vi "Periodic Tasks.vi"(8 "error in":errorcluster) -> ()   [LabVIEW 2012]
doc: "This VI runs in parallel to other tasks. It can contain as many user-defined periodic loops as you need. These can carry out PID or other sorts of timed response."
uses:
  <vilib>/Rock Robotics/WPI/DriverStation/DriverStationLCD/WPI_DriverStationLCDLCDLine.ctl
  <vilib>/Rock Robotics/SystemInterfaces/Utilities/FPGA_UtilitiesLED Source.ctl
  <vilib>/Rock Robotics/SystemInterfaces/Utilities/FPGA_UtilitiesLED State.ctl
  Robot Global Data.vi
  <vilib>/Rock Robotics/Network Tables/SD Write Boolean.vi
  <vilib>/Rock Robotics/Network Tables/SD Write Number.vi
  <vilib>/Rock Robotics/WPI/Solenoid/Deprecated/WPI_SolenoidSetBool.vi
  <vilib>/Rock Robotics/WPI/Solenoid/Deprecated/WPI_SolenoidGetBool.vi
  <vilib>/Rock Robotics/WPI/Compressor/WPI_CompressorGetSetRefNum.vi
  <vilib>/Rock Robotics/SystemInterfaces/Typedef/FPGA_TypedefAnalogModule.ctl
panel:
  out "Value":bool
  out "Up?":bool
  in  "Holding Force":dbl=0.75
  in  "Desired Speed":dbl=9500.0
  in  "Cam Speed":dbl=1.0
  out "Up to Speed?":bool
  in  "Minimum Speed":dbl=9500.0
  in  "Low Stop-Band":dbl=6.0
  in  "Scalar Multiplier":dbl=0.08
  in  "High Stop-Band":dbl=1.5
  in  "In Deadband Strength":dbl=0.5
  in  "Angle Based Deadband":dbl=7.0
  in  "PID Vision gains":T1={"proportional gain (Kc)"=1.1, "integral time (Ti, min)"=0.0, "derivative time (Td, min)"=0.0}
  in  "PID gains":T1={"proportional gain (Kc)"=0.165, "integral time (Ti, min)"=0.0, "derivative time (Td, min)"=0.0}
  in  "Teleop Vision Offset":dbl=-0.62
  in  "Autonomous Vision Offset":dbl=-0.505
  out "RPM":dbl
  in  "Voltage Adjustment":dbl=12.0
  out "Adjusted For Voltage":dbl
  out "robot battery voltage":dbl
  out "Shooter Rotation Angle":dbl
  in  "OversampleBits":u8=1
  in  "Update Averaging And Stuff":bool
  in  "AverageBits":u8
  in  "Samples Per Second":dbl
  in  "Update Sampling Rate":bool
  # "In Automatic Mode, the hopper runs unless all beam sensors are tripped. This needs refining-\nit drains batterey. Once we figure out how to best control the shooter, we can tell it to run when \nwe want to intake from the feeder station and when we want to shoot and have a fourth disk still in the belts."
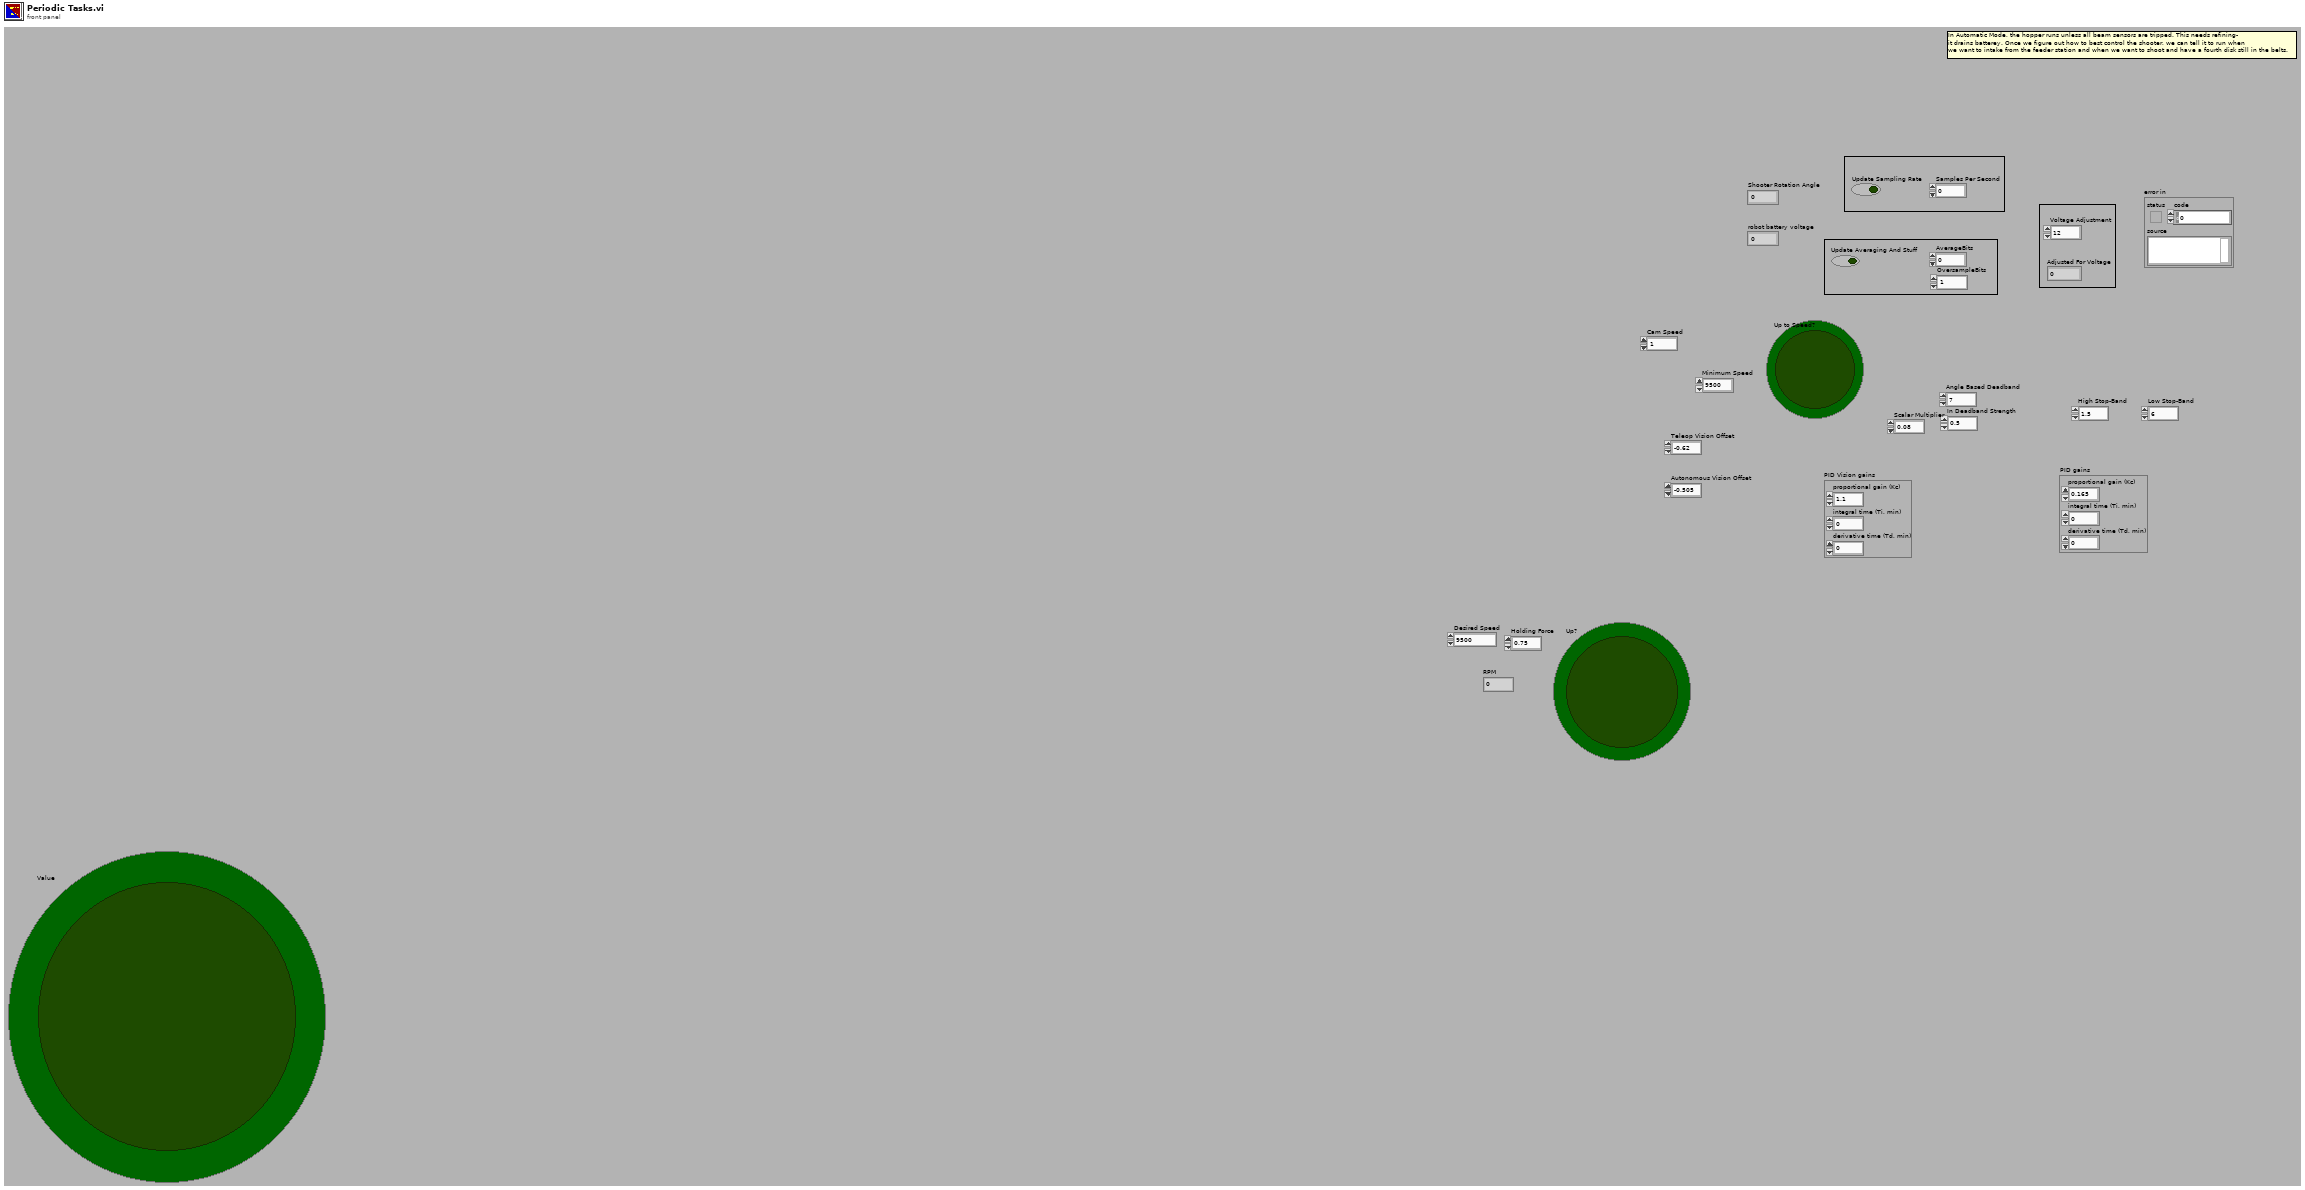
[diagram p1: front panel]
types:
  T1 = cluster{"proportional gain (Kc)":dbl, "integral time (Ti, min)":dbl, "derivative time (Td, min)":dbl}
  T2 = typedef "WPI_AnalogChannelDevRef.ctl" = cluster{"DevStatus":errorcluster, "Analog Module":T3, "Analog Channel":T4}
  T3 = typedef "FPGA_TypedefAnalogModule.ctl" = enum16{"Analog Module 1", "Analog Module 2"}
  T4 = typedef "FPGA_AIChannel.ctl" = enum8{"AI 1", "AI 2", "AI 3", "AI 4", "AI 5", "AI 6", "AI 7", "AI 8", "Invalid"}
  T5 = typedef "WPI_CounterDevRef.ctl" = cluster{"DevStatus":errorcluster, "CntIndex":T6}
  T6 = typedef "FPGA_CounterCtrSystemIndex.ctl" = enum8{"Ctr 0", "Ctr 1", "Ctr 2", "Ctr 3", "Ctr 4", "Ctr 5", "Ctr 6", "Ctr 7", "Invalid"}
  T7 = typedef "FPGA_UtilitiesLED State.ctl" = enum16{"Off", "On", "Toggle"}
  T8 = typedef "FPGA_UtilitiesLED Source.ctl" = enum16{"User LED", "FPGA LED"}
  T9 = typedef "WPI_DriverStationLCDLCDLine.ctl" = enum16{"Main - Line 1", "User - Line 2", "User - Line 3", "User - Line 4", "User - Line 5", "User - Line 6"}
  T10 = typedef "WPI_CompressorDevRef.ctl" = cluster{"DevStatus":errorcluster, "DigitalInputDevRef":T11, "RelayDevRef":T14}
  T11 = typedef "WPI_DigitalInputDevRef.ctl" = cluster{"DevStatus":errorcluster, "DIO Channel":T12, "Digital Module":T13}
  T12 = typedef "FPGA_DIOChannel.ctl" = enum8{"DIO 1", "DIO 2", "DIO 3", "DIO 4", "DIO 5", "DIO 6", "DIO 7", "DIO 8", "DIO 9", "DIO 10", "DIO 11", "DIO 12", "DIO 13", "DIO 14", "Invalid"}
  T13 = typedef "FPGA_TypedefDigitalModule.ctl" = enum16{"Digital Module 1", "Digital Module 2"}
  T14 = typedef "WPI_RelayDevRef.ctl" = cluster{"DevStatus":errorcluster, "Relay Channel":T15, "Digital Module":T13, "Relay Direction":T16}
  T15 = typedef "FPGA_DIORelayChannel.ctl" = enum8{"Relay 1", "Relay 2", "Relay 3", "Relay 4", "Relay 5", "Relay 6", "Relay 7", "Relay 8", "Invalid"}
  T16 = typedef "WPI_RelayDirection.ctl" = enum16{"Both directions", "Forward only", "Reverse only"}
  T17 = typedef "WPI_SolenoidDevRef.ctl" = cluster{"DevStatus":errorcluster, "Solenoid Module":T18, "Forward Solenoid Channel":T19, "Reverse Solenoid Channel":T19}
  T18 = typedef "FPGA_TypedefSolenoidModule.ctl" = enum16{"Solenoid Module 1", "Solenoid Module 2"}
  T19 = typedef "WPI_SolenoidChannel.ctl" = enum8{"Solenoid 1", "Solenoid 2", "Solenoid 3", "Solenoid 4", "Solenoid 5", "Solenoid 6", "Solenoid 7", "Solenoid 8", "Invalid"}
  T20 = typedef "WPI_MotorControlDeviceRef.ctl" = cluster{"DeviceStatus":errorcluster, "Type":enum16{"PWM", "CAN"}, "PWM":cluster{"Digital Module":T13, "PWM Channel":T21, "DeadBand":T22}, "CAN":cluster{"Device Number":u8, "Control Mode":T23, "Semaphore":T24, "Max Vout":dbl}, "Invert":bool, "TransformRef":T25, "InvTransformRef":T25}
  T21 = typedef "FPGA_DIOPWMChannel.ctl" = enum8{"PWM 1", "PWM 2", "PWM 3", "PWM 4", "PWM 5", "PWM 6", "PWM 7", "PWM 8", "PWM 9", "PWM 10", "Invalid"}
  T22 = typedef "WPI_PWMDeadband.ctl" = cluster{"Name":string, "maxPositivePwm":i32, "minPositivePwm":i32, "centerPwm":i32, "maxNegativePwm":i32, "minNegativePwm":i32, "angularRange":u16}
  T23 = typedef "WPI_CANJaguar_ControlMode.ctl" = enum8{"Percent VBus", "Current", "Speed", "Position", "Voltage"}
  T24 = typedef "Semaphore RefNum" = refnum<k1>
  T25 = typedef "WPI_PWMTransform_ConPane.ctl" = refnum<vi>
  T26 = typedef "WPI_DriverStationRobotMode2.ctl" = enum16{"Autonomous Disabled", "Autonomous Enabled", "Teleop Disabled", "Teleop Enabled", "Timeout", "Finish", "Test Disabled", "Test Enabled"}
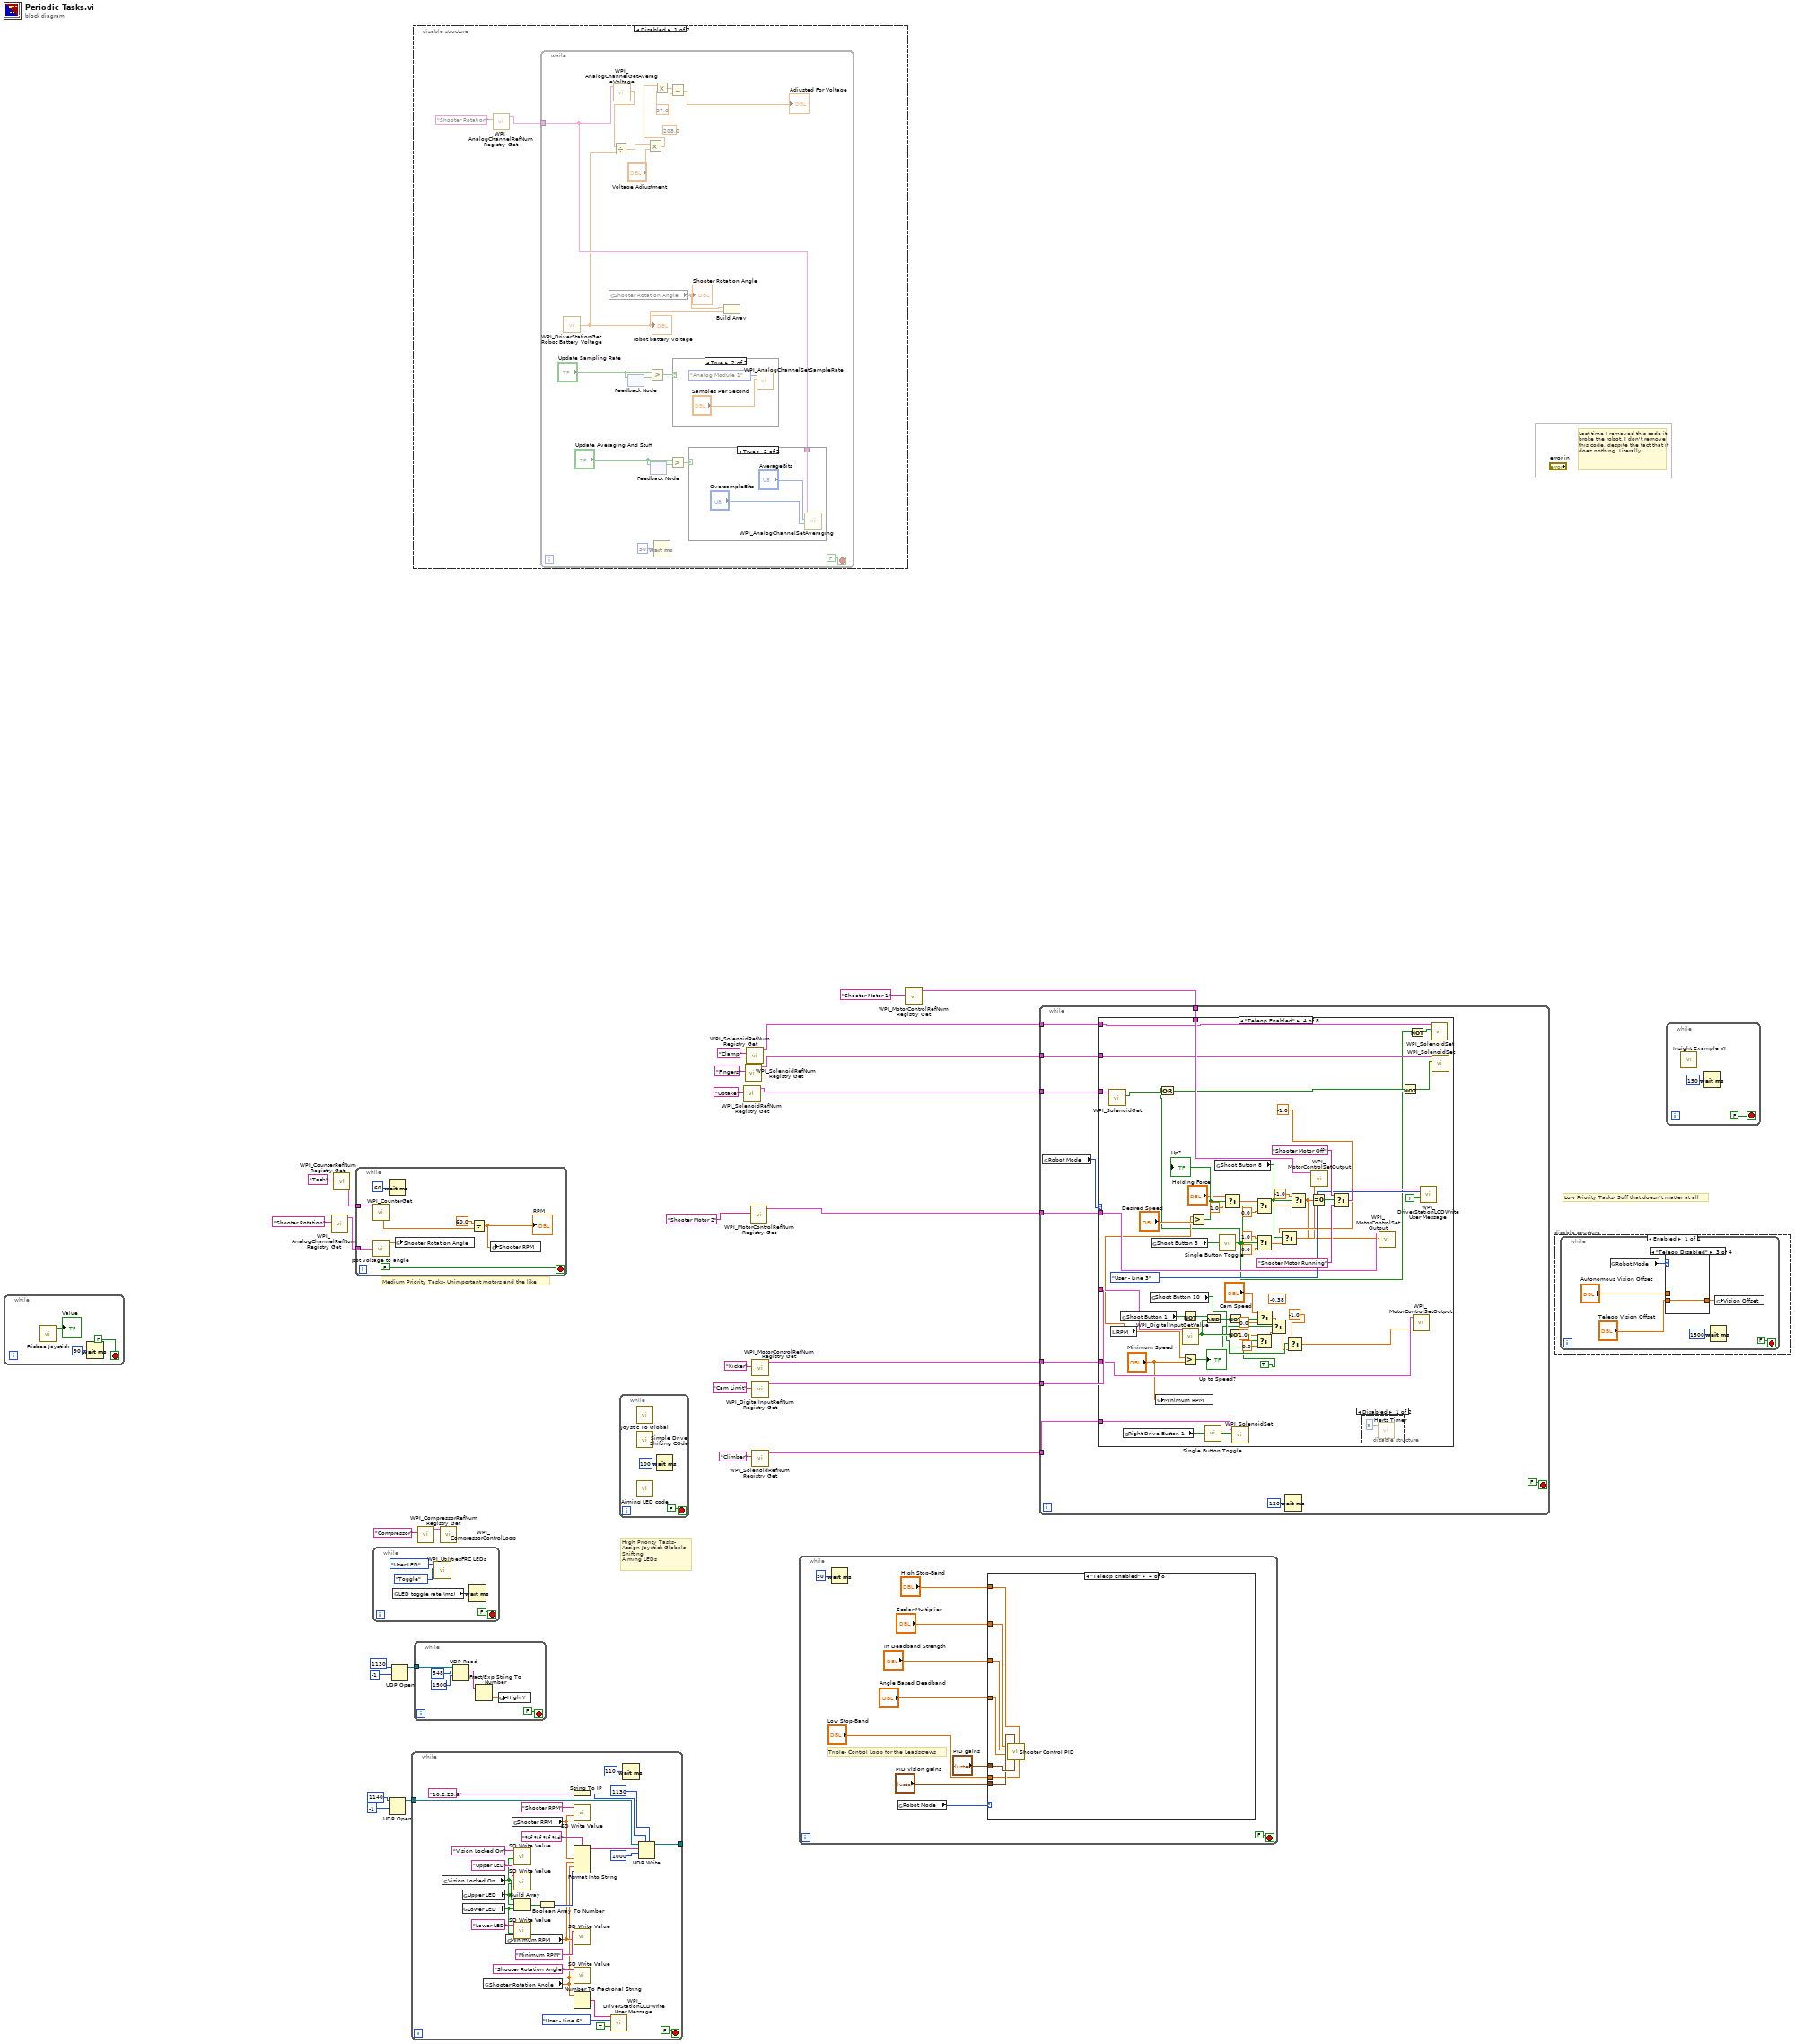
[diagram p0: block diagram]
diagram:
  # "Low Priority Tasks- Suff that doesn't matter at all"
  # "Medium Priority Tasks- Unimportant motors and the like"
  # "High Priority Tasks-\nAssign Joystick Globals\nShifting\nAiming LEDs"
  # "Last time I removed this code it broke the robot. I don't remove this code, despite the fact that it does nothing. Literally."
  n1 = while {
    stop <- FALSE stop-if-true
    n2 = call "Frisbee Joystick.vi"() -> ("Value"=→"Value":bool)  [unwired: 11 in]
    n3 = Wait (ms)(milliseconds to wait=u32 90) -> ()  [unwired: 1 out]
  }
  n4 = call <vilib>:"WPI_AnalogChannelRefNum Registry Get.vi"("refnum name"="Shooter Rotation") -> ("AIDeviceRef"=w22:T2)  [unwired: 9 in, 1 out]
  n5 = call <vilib>:"WPI_CounterRefNum Registry Get.vi"("refnum name"="Tach" ("Tach")) -> ("CounterDevRef"=w20:T5)  [unwired: 9 in, 1 out]
  n6 = while {
    tunnel: w22 -> [w37]
    tunnel: w20 -> [w36]
    stop <- FALSE stop-if-true
    n7 = call <vilib>:"WPI_CounterGet.vi"("CounterDevRef in"=w36) -> ("Period (sec)"=w34:dbl)  [unwired: 5 in, 5 out]
    n8 = call "pot voltage to angle.vi"("AIDeviceRef"=w37) -> ("Average Angle"=w38:dbl)  [unwired: 2 out]
    n9 = Wait (ms)(milliseconds to wait=u32 60) -> ()  [unwired: 1 out]
    n10 = global write "Robot Global Data.vi" "Shooter Rotation Angle"(w38) -> ()
    n11 = Divide(x=60.0, y=w34) -> (x/y=w32:dbl)
    "RPM" <- w32
    n12 = global write "Robot Global Data.vi" "Shooter RPM"(w32) -> ()
  }
  n13 = while {
    stop <- FALSE stop-if-true
    n14 = global read "Robot Global Data.vi" "LED toggle rate (ms)"() -> (w40:u32)
    n15 = call <vilib>:"WPI_UtilitiesFRC LEDs.vi"("State"=FPGA_UtilitiesLED_State."Toggle", "LED Type"=FPGA_UtilitiesLED_Source."User LED") -> ()  [unwired: 1 in, 9 out]
    n16 = Wait (ms)(milliseconds to wait=w40) -> ()  [unwired: 1 out]
  }
  n17 = UDP Open(9:-1 ("timeout ms (25000)"), 11:u16 1140 ("port")) -> (port=w3:refnum<k16>)  [unwired: 3 in, 2 out]
  n18 = UDP Open(9:-1 ("timeout ms (25000)"), 11:u16 1130 ("port")) -> (port=w25:refnum<k16>)  [unwired: 3 in, 2 out]
  n19 = while {
    tunnel: w3 -> [w69]
    tunnel: [w64] -> _
    stop <- FALSE stop-if-true
    n20 = global read "Robot Global Data.vi" "Vision Locked On"() -> (w50:bool)
    n21 = global read "Robot Global Data.vi" "Upper LED"() -> (w49:bool)
    n22 = global read "Robot Global Data.vi" "Lower LED"() -> (w48:bool)
    n23 = global read "Robot Global Data.vi" "Shooter Rotation Angle"() -> (w44:dbl)
    n24 = global read "Robot Global Data.vi" "Minimum RPM"() -> (w51:dbl)
    n25 = global read "Robot Global Data.vi" "Shooter RPM"() -> (w52:dbl)
    n26 = call-poly <vilib>:"SD Write Value.vi"("Boolean"=w50, "Name"="Vision Locked On") -> ()  [unwired: 8 in, 2 out]
    n27 = call-poly <vilib>:"SD Write Value.vi"("Boolean"=w49, "Name"="Upper LED") -> ()  [unwired: 8 in, 2 out]
    n28 = Build Array(w50, w49, w48) -> (w61:bool[])
    n29 = call-poly <vilib>:"SD Write Value.vi"("Boolean"=w48, "Name"="Lower LED") -> ()  [unwired: 8 in, 2 out]
    n30 = Boolean Array To Number(Boolean array=w61) -> (number=w60:u32)
    n31 = String To IP(1:"10.2.23.6" ("name")) -> (0:w68:u32)
    n32 = call-poly <vilib>:"SD Write Value.vi"("Numeric"=w52, "Name"="Shooter RPM") -> ()  [unwired: 8 in, 2 out]
    n33 = Format Into String(format string="%f %f %f %d", w52, w51, w44, w60) -> (resulting string=w62:string)  [unwired: 2 in, 1 out]
    n34 = call-poly <vilib>:"SD Write Value.vi"("Numeric"=w51, "Name"="Minimum RPM") -> ()  [unwired: 8 in, 2 out]
    n35 = call-poly <vilib>:"SD Write Value.vi"("Numeric"=w44, "Name"="Shooter Rotation Angle") -> ()  [unwired: 8 in, 2 out]
    n36 = Number To Fractional String(number=w44) -> (F-format string=w45:string)  [unwired: 3 in]
    n37 = call <vilib>:"WPI_DriverStationLCDWrite User Message.vi"("line text"=w45, "line"=WPI_DriverStationLCDLCDLine."User - Line 6", "clear line before write (T)"=TRUE) -> ()  [unwired: 12 in, 1 out]
    n38 = Wait (ms)(milliseconds to wait=u32 110) -> ()  [unwired: 1 out]
    n39 = UDP Write(address=w68, port or service name=u16 1130, connection ID=w69, data in=w62, 9:1000 ("timeout ms (25000)")) -> (3:w64:refnum<k16>)  [unwired: 1 in, 1 out]
  }
  n40 = disable-structure shown="Disabled" {
    frame Disabled {
      n41 = call <vilib>:"WPI_AnalogChannelRefNum Registry Get.vi"("refnum name"="Shooter Rotation") -> ("AIDeviceRef"=w71:T2)  [unwired: 9 in, 1 out]
      n42 = while {
        tunnel: w71 -> [w78]
        stop <- FALSE stop-if-true
        n43 = call <vilib>:"WPI_DriverStationGet Robot Battery Voltage.vi"() -> ("robot battery voltage"=w76:dbl)  [unwired: 14 in, 1 out]
        "robot battery voltage" <- w76
        n44 = global read "Robot Global Data.vi" "Shooter Rotation Angle"() -> (w84:dbl)
        "Shooter Rotation Angle" <- w84
        n45 = call <vilib>:"WPI_AnalogChannelGetAverageVoltage.vi"("AIDeviceRef"=w78) -> ("Voltage"=w77:dbl)  [unwired: 8 in, 2 out]
        n46 = Divide(x=w77, y=w76) -> (x/y=w75:dbl)
        n47 = feedback-in #1("Update Sampling Rate") -> ()
        n48 = feedback #1() -> (w90:bool)  [unwired: 1 in]
        n49 = Multiply(x=w75, y="Voltage Adjustment") -> (x*y=w73:dbl)
        n50 = Greater?(x="Update Sampling Rate", y=w90) -> (0:w89:bool)
        n51 = feedback #2() -> (w87:bool)  [unwired: 1 in]
        n52 = feedback-in #2("Update Averaging And Stuff") -> ()
        n53 = Wait (ms)(milliseconds to wait=u32 50) -> ()  [unwired: 1 out]
        n54 = Multiply(x=w73, y=57.0 ("X")) -> (x*y=w82:dbl)
        n55 = Greater?(x="Update Averaging And Stuff", y=w87) -> (0:w88:bool)
        n56 = Subtract(x=w82, y=208.0 ("-")) -> (x-y=→"Adjusted For Voltage":dbl)
        n57 = case shown="True" w89 {
          frame False {
          }
          frame True {
            n58 = call <vilib>:"WPI_AnalogChannelSetSampleRate.vi"("Samples Per Second"="Samples Per Second", "Analog Module (Module 1)"=FPGA_TypedefAnalogModule."Analog Module 1") -> ()  [unwired: 8 in, 2 out]
          }
        }
        n59 = case shown="True" w88 {
          tunnel: w78 -> [_ w93]
          frame False {
          }
          frame True {
            n60 = call <vilib>:"WPI_AnalogChannelSetAveraging.vi"("OversampleBits"="OversampleBits", "AverageBits"="AverageBits", "AIDeviceRef"=w93) -> ()  [unwired: 7 in, 2 out]
          }
        }
        n61 = Build Array(w84, w76) -> (w83:dbl[])
      }
    }
    frame Enabled {
    }
  }
  n62 = while {
    tunnel: w25 -> [w103]
    stop <- FALSE stop-if-true
    n63 = UDP Read(connection ID=w103, max size (548)=548, timeout ms (25000)=1500) -> (data out=w98:string)  [unwired: 1 in, 4 out]
    n64 = Fract/Exp String To Number(string=w98) -> (number=w99:dbl)  [unwired: 3 in, 1 out]
    n65 = global write "Robot Global Data.vi" "High Y"(w99) -> ()
  }
  n66 = call <vilib>:"WPI_CompressorRefNum Registry Get.vi"("refnum name"="Compressor") -> ("CompressorDevRef"=w28:T10)  [unwired: 9 in, 1 out]
  n67 = call <vilib>:"WPI_CompressorControlLoop.vi"("CompressorDevRef"=w28) -> ()  [unwired: 11 in]
  n68 = while {
    stop <- FALSE stop-if-true
    n69 = call "Joystic To Global.vi"() -> ()  [unwired: 12 in]
    n70 = call "Simple Drive Shifting COde.vi"() -> ()  [unwired: 12 in]
    n71 = call "Aiming LED code.vi"() -> ()  [unwired: 12 in]
    n72 = Wait (ms)(milliseconds to wait=u32 100) -> ()  [unwired: 1 out]
  }
  n73 = call <vilib>:"WPI_SolenoidRefNum Registry Get.vi"("refnum name"="Uptake") -> ("SolenoidDevRef"=w8:T17)  [unwired: 9 in, 1 out]
  n74 = call <vilib>:"WPI_SolenoidRefNum Registry Get.vi"("refnum name"="Fingers") -> ("SolenoidDevRef"=w6:T17)  [unwired: 9 in, 1 out]
  n75 = call <vilib>:"WPI_SolenoidRefNum Registry Get.vi"("refnum name"="Clamp") -> ("SolenoidDevRef"=w7:T17)  [unwired: 9 in, 1 out]
  n76 = call <vilib>:"WPI_MotorControlRefNum Registry Get.vi"("refnum name"="Shooter Motor 2") -> ("MotorControlDevRef"=w10:T20)  [unwired: 9 in, 1 out]
  n77 = call <vilib>:"WPI_MotorControlRefNum Registry Get.vi"("refnum name"="Kicker") -> ("MotorControlDevRef"=w14:T20)  [unwired: 9 in, 1 out]
  n78 = call <vilib>:"WPI_DigitalInputRefNum Registry Get.vi"("refnum name"="Cam Limit") -> ("DigitalInputDevRef"=w16:T11)  [unwired: 9 in, 1 out]
  n79 = call <vilib>:"WPI_SolenoidRefNum Registry Get.vi"("refnum name"="Climber") -> ("SolenoidDevRef"=w18:T17)  [unwired: 9 in, 1 out]
  n80 = while {
    stop <- FALSE stop-if-true
    # "Triple- Control Loop for the Leadscrews"
    n81 = Wait (ms)(milliseconds to wait=u32 50) -> ()  [unwired: 1 out]
    n82 = global read "Robot Global Data.vi" "Robot Mode"() -> (w106:T26)
    n83 = case shown="\"Teleop Enabled\"" w106 {
      tunnel: "PID gains" -> [_ _ _ w122 _ _ _ _]
      tunnel: "PID Vision gains" -> [_ _ _ w121 _ _ _ _]
      tunnel: "Angle Based Deadband" -> [_ _ _ w120 _ _ _ _]
      tunnel: "High Stop-Band" -> [_ _ _ w119 _ _ _ _]
      tunnel: "In Deadband Strength" -> [_ _ _ w118 _ _ _ _]
      tunnel: "Low Stop-Band" -> [_ _ _ w117 _ _ _ _]
      tunnel: "Scalar Multiplier" -> [_ _ _ w116 _ _ _ _]
      frame "Autonomous Disabled", Default {
      }
      frame "Autonomous Enabled" {
      }
      frame "Teleop Disabled" {
      }
      frame "Teleop Enabled" {
        n84 = call "Shooter Control PID.vi"("Low Stop-Band"=w117, "High Stop-Band"=w119, "PID gains"=w122, "PID Vision gains"=w121, "Angle Based Deadband"=w120, "In Deadband Strength"=w118, "y"=w116) -> ()  [unwired: 3 in, 2 out]
      }
      frame "Timeout" {
      }
      frame "Finish" {
      }
      frame "Test Disabled" {
      }
      frame "Test Enabled" {
      }
    }
  }
  n85 = call <vilib>:"WPI_MotorControlRefNum Registry Get.vi"("refnum name"="Shooter Motor 1") -> ("MotorControlDevRef"=w12:T20)  [unwired: 9 in, 1 out]
  n86 = while {
    tunnel: w18 -> [w132]
    tunnel: w16 -> [w131]
    tunnel: w14 -> [w130]
    tunnel: w12 -> [w129]
    tunnel: w10 -> [w128]
    tunnel: w8 -> [w127]
    tunnel: w7 -> [w126]
    tunnel: w6 -> [w125]
    stop <- FALSE stop-if-true
    n87 = global read "Robot Global Data.vi" "Robot Mode"() -> (w124:T26)
    n88 = case shown="\"Teleop Enabled\"" w124 {
      tunnel: w132 -> [_ _ _ w178 _ _ _ _]
      tunnel: w131 -> [_ _ _ w177 _ _ _ _]
      tunnel: w130 -> [_ _ _ w176 _ _ _ _]
      tunnel: w129 -> [_ _ _ w174 _ _ _ _]
      tunnel: w128 -> [_ _ _ w173 _ _ _ _]
      tunnel: w127 -> [_ _ _ w161 _ _ _ _]
      tunnel: w126 -> [_ _ _ w160 _ _ _ _]
      tunnel: w125 -> [_ _ _ w159 _ _ _ _]
      frame "Autonomous Disabled", Default {
      }
      frame "Autonomous Enabled" {
      }
      frame "Teleop Disabled" {
      }
      frame "Teleop Enabled" {
        (unwired) -0.38 ("t")
        n89 = call-poly <vilib>:"WPI_SolenoidGet.vi"("SolenoidDevRef"=w161) -> ("Value"=w157:bool)  [unwired: 8 in, 2 out]
        n90 = local read "RPM"() -> (w146:dbl)
        n91 = global read "Robot Global Data.vi" "Shoot Button 1"() -> (w175:bool)
        n92 = global read "Robot Global Data.vi" "Right Drive Button 1"() -> (w180:bool)
        n93 = global read "Robot Global Data.vi" "Shoot Button 10"() -> (w154:bool)
        n94 = global read "Robot Global Data.vi" "Shoot Button 3"() -> (w181:bool)
        n95 = global write "Robot Global Data.vi" "Minimum RPM"("Minimum Speed") -> ()
        n96 = Not(x=w175) -> (.not. x?=w172:bool)
        n97 = Greater?(x=w146, y="Minimum Speed") -> (0:→"Up to Speed?":bool)
        n98 = call <vilib>:"WPI_DigitalInputGetValue.vi"("DigitalInputDevRef"=w177) -> ("Value"=w171:bool)  [unwired: 8 in, 2 out]
        n99 = Greater?(x=w146, y="Desired Speed") -> (0:w150:bool)
        "Up?" <- w150
        n100 = call "Single Button Toggle.vi"("Shoot Button 3"=w180) -> ("Boolean"=w179:bool)
        n101 = And(x=w172, y=w171) -> (x .and. y?=w170:bool)
        n102 = global read "Robot Global Data.vi" "Shoot Button 8"() -> (w140:bool)
        n103 = call "Single Button Toggle.vi"("Shoot Button 3"=w181) -> ("Boolean"=w143:bool)
        n104 = Or(x=w143, y=w157) -> (x .or. y?=w156:bool)
        n105 = Select(t="Holding Force", s=w150, f=1.0 ("Shooter Speed")) -> (s? t:f=w148:dbl)
        n106 = Not(x=w170) -> (.not. x?=w169:bool)
        n107 = Not(x=w171) -> (.not. x?=w167:bool)
        n108 = call-poly <vilib>:"WPI_SolenoidSet.vi"("Value"=w179, "SolenoidDevRef"=w178) -> ()  [unwired: 8 in, 2 out]
        n109 = Select(t=w148, s=w143, f=0.0) -> (s? t:f=w183:dbl)
        n110 = Select(t=1.0, s=w143, f=0.0) -> (s? t:f=w141:dbl)
        n111 = Select(t=1.0, s=w167, f=0.0) -> (s? t:f=w166:dbl)
        n112 = Select(t="Cam Speed", s=w169, f=0.0) -> (s? t:f=w168:dbl)
        n113 = Select(t=w168, s=TRUE, f=w166) -> (s? t:f=w153:dbl)
        n114 = Select(t=-1.0, s=w140, f=w141) -> (s? t:f=w139:dbl)
        n115 = Select(t=-1.0, s=w154, f=w153) -> (s? t:f=w137:dbl)
        n116 = Select(t=-1.0, s=w140, f=w183) -> (s? t:f=w138:dbl)
        n117 = Equal To 0?(x=w138) -> (x = 0?=w184:bool)
        n118 = call <vilib>:"WPI_MotorControlSetOutput.vi"("Output"=w139, "MotorControlDevRef"=w174) -> ()  [unwired: 7 in, 3 out]
        n119 = Select(t="Shooter Motor Off", s=w184, f="Shooter Motor Running" ("refnum name")) -> (s? t:f=w189:string)
        n120 = disable-structure shown="Disabled" {
          frame Disabled {
            n121 = call "Hertz Timer.vi"("How many times per second do we want the loop to run?"=8) -> ()  [unwired: 11 in]
          }
          frame Enabled {
          }
        }
        n122 = call <vilib>:"WPI_MotorControlSetOutput.vi"("Output"=w138, "MotorControlDevRef"=w173) -> ()  [unwired: 7 in, 3 out]
        n123 = Not(x=w156) -> (.not. x?=w155:bool)
        n124 = Not(x=w143) -> (.not. x?=w158:bool)
        n125 = call <vilib>:"WPI_MotorControlSetOutput.vi"("Output"=w137, "MotorControlDevRef"=w176) -> ()  [unwired: 7 in, 3 out]
        n126 = call <vilib>:"WPI_DriverStationLCDWrite User Message.vi"("line text"=w189, "line"=WPI_DriverStationLCDLCDLine."User - Line 3", "clear line before write (T)"=TRUE) -> ()  [unwired: 12 in, 1 out]
        n127 = call-poly <vilib>:"WPI_SolenoidSet.vi"("Value"=w158, "SolenoidDevRef"=w160) -> ()  [unwired: 8 in, 2 out]
        n128 = call-poly <vilib>:"WPI_SolenoidSet.vi"("Value"=w155, "SolenoidDevRef"=w159) -> ()  [unwired: 8 in, 2 out]
      }
      frame "Timeout" {
      }
      frame "Finish" {
      }
      frame "Test Disabled" {
      }
      frame "Test Enabled" {
      }
    }
    n129 = Wait (ms)(milliseconds to wait=u32 120) -> ()  [unwired: 1 out]
  }
  n130 = disable-structure shown="Enabled" {
    frame Enabled {
      n131 = while {
        stop <- FALSE stop-if-true
        n132 = global read "Robot Global Data.vi" "Robot Mode"() -> (w197:T26)
        n133 = case shown="\"Teleop Disabled\"" w197 {
          tunnel: [w198 w199 w200 w201] -> w195
          tunnel: "Teleop Vision Offset" -> [_ _ w200 w201]
          tunnel: "Autonomous Vision Offset" -> [w198 w199 _ _]
          frame "Autonomous Disabled", Default {
          }
          frame "Autonomous Enabled" {
          }
          frame "Teleop Disabled" {
          }
          frame "Teleop Enabled" {
          }
        }
        n134 = Wait (ms)(milliseconds to wait=u32 1500) -> ()  [unwired: 1 out]
        n135 = global write "Robot Global Data.vi" "Vision Offset"(w195) -> ()
      }
    }
  }
  n136 = while {
    stop <- FALSE stop-if-true
    n137 = call "Insight Example VI.vi"() -> ()  [unwired: 1 in]
    n138 = Wait (ms)(milliseconds to wait=u32 150) -> ()  [unwired: 1 out]
  }
